vi "niRFUtil CONV dBm to 1 Ohm Watt (real scalar).vi"(7 "Real Scalar (dBm)":sgl format="%.2f") -> (8 "Real Scalar (W)":sgl format="%.2f")   [LabVIEW 2015, in "niRFUtil.lvlib"]
doc: "(c) Copyright 2006, National Instruments, Inc. This VI may not be duplicated, sold, or distributed without written consent from National Instruments."
uses:
  niRFUtil.lvlib
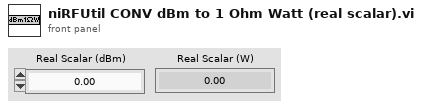
[diagram p1: front panel]
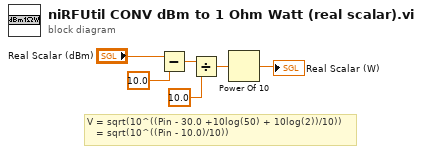
[diagram p0: block diagram]
diagram:
  # "V = sqrt(10^((Pin - 30.0 +10log(50) + 10log(2))/10))\n   = sqrt(10^((Pin - 10.0)/10))"
  n1 = Subtract(x="Real Scalar (dBm)", y=sgl 10.0) -> (x-y=w6:sgl)
  n2 = Divide(x=w6, y=sgl 10.0) -> (x/y=w4:sgl)
  n3 = Power Of 10(x=w4) -> (10^x=→"Real Scalar (W)":sgl)
